vi "Daqmx config.vi"(7 "FV":T5, 8 "error in (no error)":errorcluster) -> (0 "error out":errorcluster, 1 "CI Settings":T1, 2 "CO Settings":T2, 3 "AI Settings":T3)   [LabVIEW 2017]
uses:
  Controls/FV_Daqmx config.ctl
  Share data/Default volues.vi
panel:
  in  "Cancel":bool
  in  "OK":bool
  in  "Tab Control":T4(tab)
  in  "Digital Start Trigger Edge":i32(ring)=10280 caption="Edge" items=["Rising"=10280, "Falling"=10171]
  in  "Digital Start Trigger Source":tag="/Dev1/PFI0" caption="Trigger Source"
  in  "Terminal Configuration":i32(ring)=-1 items=["default"=-1, "RSE"=10083, "NRSE"=10078, "Differential"=10106, "Pseudodifferential"=12529]
  in  "Max Voltage":dbl=5.0
  in  "Min Voltage":dbl=-5.0
  in  "AI Channel":tag="Dev1/ai0"
  in  "low ticks":u32=100
  in  "high ticks":u32=100
  in  "source of ticks":tag="OnboardClock"
  in  "Output Terminal":tag="/Dev1/PFI12"
  in  "CO_Counter":tag="Dev1/ctr0"
  in  "Z Index Terminal":tag="PFI9"
  in  "Z Index Enable":bool
  in  "Pulses Per Revolution":u32=24
  in  "B Input Terminal":tag="PFI10"
  in  "A Input Terminal":tag="PFI8"
  in  "CI_Counter":tag="Dev1/ctr0"
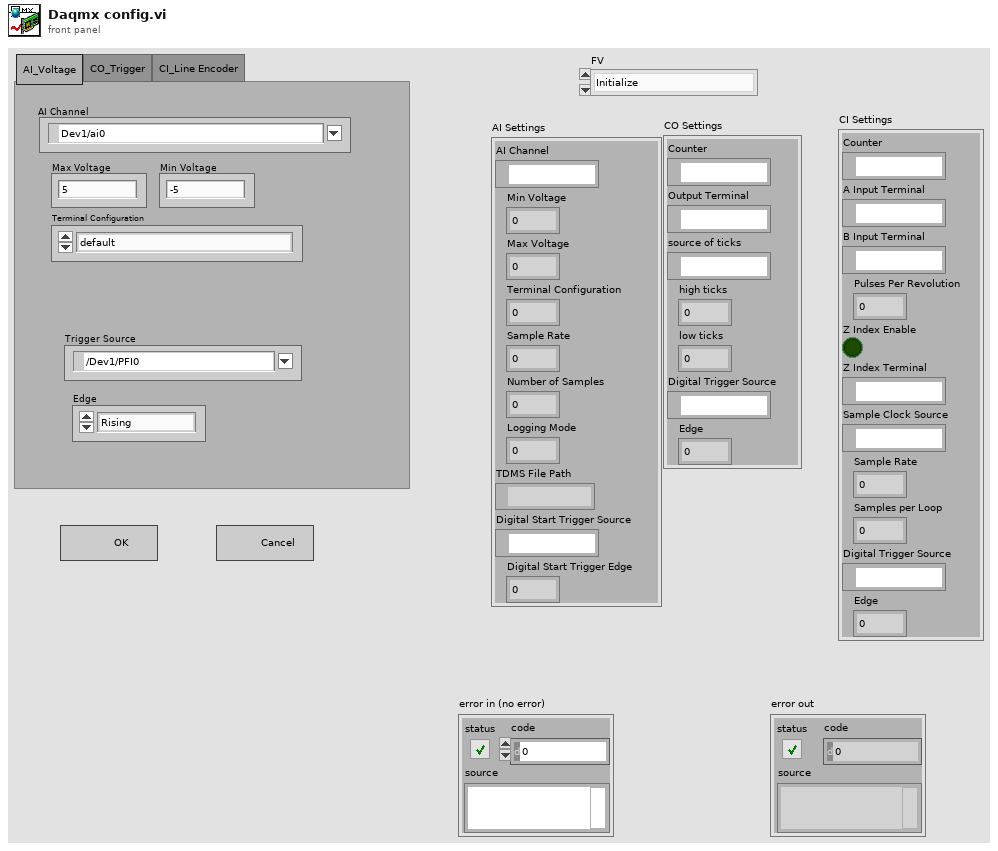
[diagram p1: front panel]
types:
  T1 = cluster{"Counter":tag, "A Input Terminal":tag, "B Input Terminal":tag, "Pulses Per Revolution":u32, "Z Index Enable":bool, "Z Index Terminal":tag, "Sample Clock Source":tag, "Sample Rate":dbl, "Samples per Loop":i32, "Digital Trigger Source":tag, "Edge":i32}
  T2 = cluster{"Counter":tag, "Output Terminal":tag, "source of ticks":tag, "high ticks":u32, "low ticks":u32, "Digital Trigger Source":tag, "Edge":i32}
  T3 = cluster{"AI Channel":tag, "Min Voltage":dbl, "Max Voltage":dbl, "Terminal Configuration":i32, "Sample Rate":dbl, "Number of Samples":i32, "Logging Mode":i32, "TDMS File Path":path, "Digital Start Trigger Source":tag, "Digital Start Trigger Edge":i32}
  T4 = enum32{"AI_Voltage", "CO_Trigger", "CI_Line Encoder"}
  T5 = typedef "FV_Daqmx config.ctl" = enum16{"Initialize", "SetDefault", "UI_input", "GetAI", "GetCO", "GetCI"}
  T6 = cluster{"AI Settings":cluster{"AI Channel":tag, "Min Voltage":dbl, "Max Voltage":dbl, "Terminal Configuration":i32, "Sample Rate":dbl, "Number of Samples":i32, "Logging Mode":i32, "TDMS File Path":path, "Digital Start Trigger Source":tag, "Digital Start Trigger Edge":i32}, "CO Settings":cluster{"Counter":tag, "Output Terminal":tag, "source of ticks":tag, "high ticks":u32, "low ticks":u32, "Digital Trigger Source":tag, "Edge":i32}, "CI Settings":cluster{"Counter":tag, "A Input Terminal":tag, "B Input Terminal":tag, "Pulses Per Revolution":u32, "Z Index Enable":bool, "Z Index Terminal":tag, "Sample Clock Source":tag, "Sample Rate":dbl, "Samples per Loop":i32, "Digital Trigger Source":tag, "Edge":i32}}
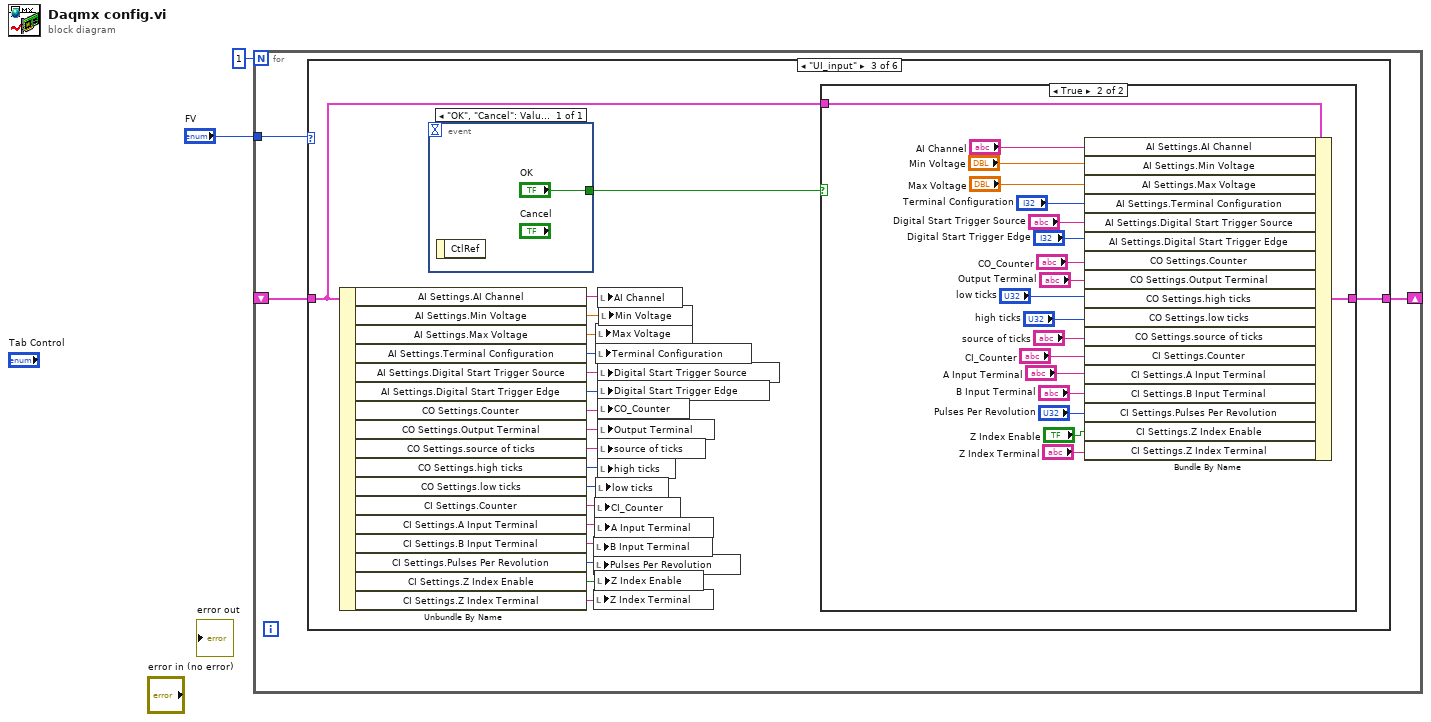
[diagram p0: block diagram]
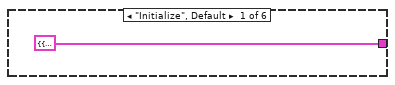
[diagram p2: hidden frame]
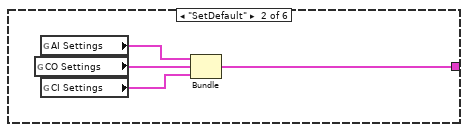
[diagram p3: hidden frame]
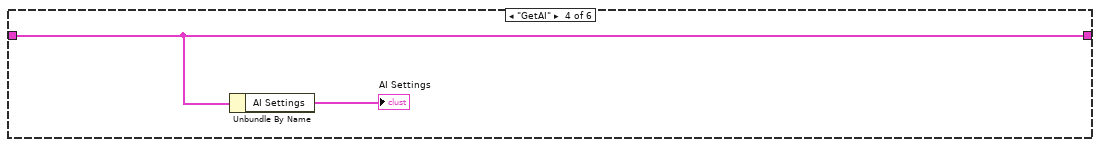
[diagram p5: hidden frame]
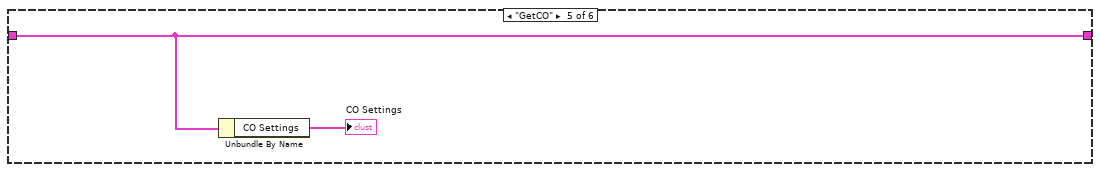
[diagram p6: hidden frame]
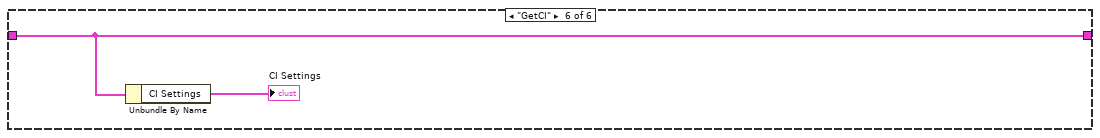
[diagram p7: hidden frame]
diagram:
  n1 = for {
    N: 1 -> [_]
    tunnel: "FV" -> [w5]
    shift-right: [w4] -> _
    shift-left: _ -> [w3]
    n2 = case shown="\"UI_input\"" w5 {
      tunnel: [T6 {"AI Settings"={"AI Channel"="", "Min Voltage"=0.0, "Max Voltage"=0.0, "Terminal Configuration"=0, "Sample Rate"=0.0, "Number of Samples"=0, "Logging Mode"=0, "TDMS File Path"=path "", "Digital Start Trigger Source"="", "Digital Start Trigger Edge"=0}, "CO Settings"={"Counter"="", "Output Terminal"="", "source of ticks"="", "high ticks"=0, "low ticks"=0, "Digital Trigger Source"="", "Edge"=0}, "CI Settings"={"Counter"="", "A Input Terminal"="", "B Input Terminal"="", "Pulses Per Revolution"=0, "Z Index Enable"=FALSE, "Z Index Terminal"="", "Sample Clock Source"="", "Sample Rate"=0.0, "Samples per Loop"=0, "Digital Trigger Source"="", "Edge"=0}} w7 w11 w53 w55 w57] -> w4
      tunnel: w3 -> [_ _ w13 w53 w55 w57]
      frame "Initialize", Default {
      }
      frame "SetDefault" {
        n3 = global read "Default volues.vi" "CO Settings"() -> (w10:T2)
        n4 = global read "Default volues.vi" "AI Settings"() -> (w9:T3)
        n5 = global read "Default volues.vi" "CI Settings"() -> (w8:T1)
        n6 = Bundle("AI Settings"=w9, "CO Settings"=w10, "CI Settings"=w8) -> (w7:T6)  [unwired: 1 in]
      }
      frame "UI_input" {
        n7 = Unbundle By Name(w13) -> ("AI Settings.AI Channel"=w30:tag, "AI Settings.Min Voltage"=w29:dbl, "AI Settings.Max Voltage"=w28:dbl, "AI Settings.Terminal Configuration"=w27:i32, "AI Settings.Digital Start Trigger Source"=w26:tag, "AI Settings.Digital Start Trigger Edge"=w25:i32, "CO Settings.Counter"=w24:tag, "CO Settings.Output Terminal"=w23:tag, "CO Settings.source of ticks"=w22:tag, "CO Settings.high ticks"=w21:u32, "CO Settings.low ticks"=w20:u32, "CI Settings.Counter"=w19:tag, "CI Settings.A Input Terminal"=w18:tag, "CI Settings.B Input Terminal"=w17:tag, "CI Settings.Pulses Per Revolution"=w16:u32, "CI Settings.Z Index Enable"=w15:bool, "CI Settings.Z Index Terminal"=w14:tag)
        n8 = event shown="[0] \"OK\", \"Cancel\": Value Change" {
          selector: _ -> [_]
          dyn-events: _ -> [_]
          timeout: _ -> [_]
          tunnel: ["OK"] -> w12
          event "OK", "Cancel": Value Change {
            n9 = event-data() -> ()  [unwired: 1 in, 1 out]
          }
        }
        n10 = local write "B Input Terminal"(w17) -> ()
        n11 = local write "Pulses Per Revolution"(w16) -> ()
        n12 = local write "Z Index Terminal"(w14) -> ()
        n13 = local write "CI_Counter"(w19) -> ()
        n14 = local write "A Input Terminal"(w18) -> ()
        n15 = local write "Z Index Enable"(w15) -> ()
        n16 = local write "Max Voltage"(w28) -> ()
        n17 = local write "Terminal Configuration"(w27) -> ()
        n18 = local write "low ticks"(w20) -> ()
        n19 = local write "AI Channel"(w30) -> ()
        n20 = local write "Digital Start Trigger Source"(w26) -> ()
        n21 = local write "Digital Start Trigger Edge"(w25) -> ()
        n22 = local write "CO_Counter"(w24) -> ()
        n23 = local write "Output Terminal"(w23) -> ()
        n24 = local write "source of ticks"(w22) -> ()
        n25 = local write "high ticks"(w21) -> ()
        n26 = local write "Min Voltage"(w29) -> ()
        n27 = case shown="True" w12 {
          tunnel: w13 -> [w31 w50]
          tunnel: [w31 w32] -> w11
          frame False {
          }
          frame True {
            n28 = Bundle By Name(cluster=w50, "AI Settings.AI Channel"="AI Channel", "AI Settings.Min Voltage"="Min Voltage", "AI Settings.Max Voltage"="Max Voltage", "AI Settings.Terminal Configuration"="Terminal Configuration", "AI Settings.Digital Start Trigger Source"="Digital Start Trigger Source", "AI Settings.Digital Start Trigger Edge"="Digital Start Trigger Edge", "CO Settings.Counter"="CO_Counter", "CO Settings.Output Terminal"="Output Terminal", "CO Settings.high ticks"="low ticks", "CO Settings.low ticks"="high ticks", "CO Settings.source of ticks"="source of ticks", "CI Settings.Counter"="CI_Counter", "CI Settings.A Input Terminal"="A Input Terminal", "CI Settings.B Input Terminal"="B Input Terminal", "CI Settings.Pulses Per Revolution"="Pulses Per Revolution", "CI Settings.Z Index Enable"="Z Index Enable", "CI Settings.Z Index Terminal"="Z Index Terminal") -> (w32:T6)
          }
        }
      }
      frame "GetAI" {
        n29 = Unbundle By Name(w53) -> ("AI Settings"=→"AI Settings":T3)
      }
      frame "GetCO" {
        n30 = Unbundle By Name(w55) -> ("CO Settings"=→"CO Settings":T2)
      }
      frame "GetCI" {
        n31 = Unbundle By Name(w57) -> ("CI Settings"=→"CI Settings":T1)
      }
    }
  }
